vi "TCP_Test Disconnected by Peer.vi"(8 "error in":errorcluster) -> (0 "error out":errorcluster)   [LabVIEW 2013]
uses:
  <vilib>/addons/_JKI Toolkits/Caraya/classes/Assert/Assert Not Error.vi
  <vilib>/addons/_JKI Toolkits/Caraya/classes/Assert/Assert Equal Value_Variant.vi
  <vilib>/LabVIEW Open Source Project/Connection/Connection/Connection.lvclass
  source/MQTT_TCP/Connection/TCPConnection.lvclass
  <vilib>/addons/_JKI Toolkits/Caraya/classes/Test/Test.lvclass
  <vilib>/addons/_JKI Toolkits/Caraya/classes/Assert/Assert.lvclass
panel:
  out "connected":bool
  out "server connected":bool
  out "client connected":bool
  out "Comm OK":bool
  out "value":dbl
  out "Bytes":u8[](array[numeric]) format="%08b"
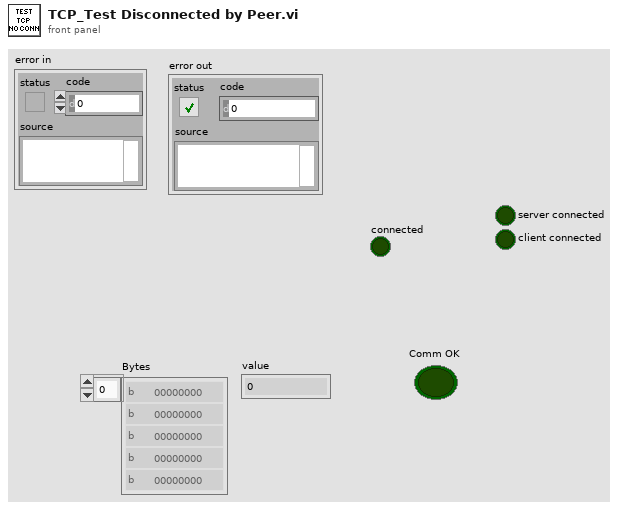
[diagram p1: front panel]
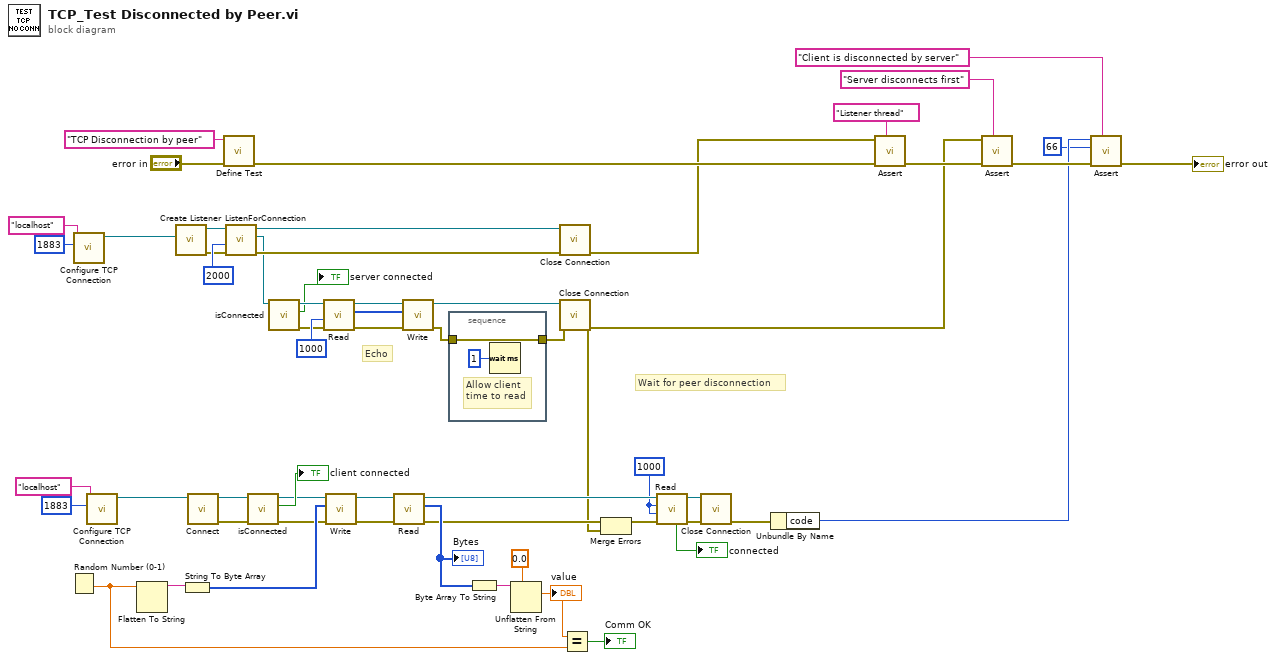
[diagram p0: block diagram]
diagram:
  w8 = 1000 ("bytes to read (100)")
  # "Wait for peer disconnection"
  # "Echo"
  n1 = Random Number (0-1)() -> (number: 0 to 1=w23:dbl)
  n2 = call "Configure TCP Connection.vi"("remote port (80)"=u16 1883, "address (localhost)"="localhost") -> ("TCPConnection"=w30:refnum<class "TCPConnection.lvclass">)  [unwired: 8 in, 1 out]
  n3 = call "Configure TCP Connection.vi"("remote port (80)"=u16 1883, "address (localhost)"="localhost") -> ("TCPConnection"=w29:refnum<class "TCPConnection.lvclass">)  [unwired: 8 in, 1 out]
  n4 = Flatten To String(anything=w23) -> (data string=w36:string)  [unwired: 3 in, 2 out]
  n5 = call <vilib>:"Create Listener.vi"("Connection Configuration"=w30) -> ("error out"=w44:errorcluster, "Listener"=w47:refnum<class "TCPConnection.lvclass">)  [unwired: 9 in]
  n6 = String To Byte Array(string=w36) -> (unsigned byte array=w35:u8[])
  n7 = call <vilib>:"Connect.vi"("Connection in"=w29) -> ("error out"=w18:errorcluster, "Connection out"=w16:refnum<class "TCPConnection.lvclass">)  [unwired: 9 in]
  n8 = call <vilib>:"Define Test.vi"("error in (no error)"="error in", "Label (VI Title)"="TCP Disconnection by peer") -> ("error out"=w57:errorcluster)  [unwired: 9 in]
  n9 = call <vilib>:"ListenForConnection.vi"("error in (no error)"=w44, "timeout (2000 ms)"=2000 ("bytes to read (100)"), "Listener"=w47) -> ("error out"=w31:errorcluster, "Connection"=w14:refnum<class "Connection.lvclass">, "Listener out"=w45:refnum<class "TCPConnection.lvclass">)  [unwired: 5 in, 1 out]
  n10 = call <vilib>:"isConnected.vi"("error in (no error)"=w18, "Connection in"=w16) -> ("error out"=w17:errorcluster, "connected"=→"client connected":bool, "Connection out"=w15:refnum<class "TCPConnection.lvclass">)  [unwired: 7 in]
  n11 = call <vilib>:"isConnected.vi"("Connection in"=w14) -> ("error out"=w12:errorcluster, "connected"=→"server connected":bool, "Connection out"=w13:refnum<class "Connection.lvclass">)  [unwired: 8 in]
  n12 = call <vilib>:"Read.vi"("error in (no error)"=w12, "timeout (2000 ms)"=1000 ("bytes to read (100)"), "TCPConnection in"=w13) -> ("error out"=w39:errorcluster, "Bytes"=w41:u8[], "TCPConnection out"=w42:refnum<class "Connection.lvclass">)  [unwired: 4 in, 2 out]
  n13 = call <vilib>:"Write.vi"("error in (no error)"=w17, "Bytes"=w35, "Connection in"=w15) -> ("error out"=w38:errorcluster, "Connection"=w40:refnum<class "TCPConnection.lvclass">)  [unwired: 7 in]
  n14 = call <vilib>:"Read.vi"("error in (no error)"=w38, "TCPConnection in"=w40) -> ("error out"=w4:errorcluster, "Bytes"=w34:u8[], "TCPConnection out"=w10:refnum<class "TCPConnection.lvclass">)  [unwired: 5 in, 2 out]
  "Bytes" <- w34
  n15 = call <vilib>:"Write.vi"("error in (no error)"=w39, "Bytes"=w41, "Connection in"=w42) -> ("error out"=w21:errorcluster, "Connection"=w37:refnum<class "Connection.lvclass">)  [unwired: 7 in]
  n16 = stacked-sequence {
    tunnel: w21 -> [w59]
    tunnel: [w59] -> w20
    frame #0 {
      # "Allow client\ntime to read"
      n17 = Wait (ms)(milliseconds to wait=u32 1) -> ()  [unwired: 1 out]
    }
  }
  n18 = Byte Array To String(unsigned byte array=w34) -> (string=w33:string)
  n19 = Unflatten From String(type=0.0, binary string=w33) -> (value=w24:dbl)  [unwired: 3 in, 2 out]
  "value" <- w24
  n20 = call <vilib>:"Close Connection.vi"("error in (no error)"=w31, "Connection in"=w45) -> ("error out"=w7:errorcluster)  [unwired: 8 in, 1 out]
  n21 = call <vilib>:"Close Connection.vi"("error in (no error)"=w20, "Connection in"=w37) -> ("error out"=w3:errorcluster)  [unwired: 8 in, 1 out]
  n22 = Equal?(x=w24, y=w23) -> (x = y?=→"Comm OK":bool)
  n23 = Merge Errors(w4, w3) -> (w2:errorcluster)
  n24 = call <vilib>:"Read.vi"("error in (no error)"=w2, "timeout (2000 ms)"=w8, "bytes to read (100)"=w8, "TCPConnection in"=w10) -> ("error out"=w5:errorcluster, "TCPConnection out"=w9:refnum<class "TCPConnection.lvclass">, "connected"=→"connected":bool)  [unwired: 3 in, 2 out]
  n25 = call <vilib>:"Close Connection.vi"("error in (no error)"=w5, "Connection in"=w9) -> ("error out"=w6:errorcluster)  [unwired: 8 in, 1 out]
  n26 = Unbundle By Name(w6) -> ("code"=w54:i32)
  n27 = call-poly <vilib>:"Assert.vi"("Label"="Listener thread" ("Label (VI Title)"), "error in (no error)"=w57, "Not Error?"=w7) -> ("error out"=w56:errorcluster)  [unwired: 8 in]
  n28 = call-poly <vilib>:"Assert.vi"("Label"="Server disconnects first" ("Label (VI Title)"), "error in (no error)"=w56, "Not Error?"=w3) -> ("error out"=w55:errorcluster)  [unwired: 8 in]
  n29 = call-poly <vilib>:"Assert.vi"("Label"="Client is disconnected by server" ("Label (VI Title)"), "error in (no error)"=w55, "Y"=66 ("code"), "X"=w54) -> ("error out"=→"error out":errorcluster)  [unwired: 7 in]
